vi "getIndex.vi"(11 "ModbusBuffer in":refnum<class "ModbusBuffer.lvclass">) -> (2 "Index":i32, 3 "ModbusBuffer out":refnum<class "ModbusBuffer.lvclass">)   [LabVIEW 2016, in "RTModbus.lvlib" / "ModbusBuffer.lvclass"]
uses:
  ModbusBuffer.lvclass
  ModbusBuffer.lvclass/ModbusBuffer.ctl
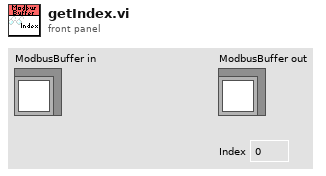
[diagram p1: front panel]
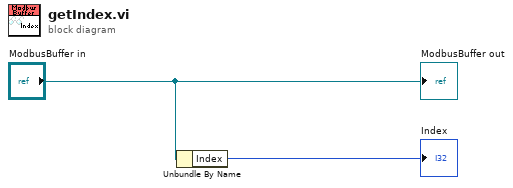
[diagram p0: block diagram]
diagram:
  n1 = Unbundle By Name("ModbusBuffer in") -> ("Index"=→"Index":i32)
  "ModbusBuffer out" <- "ModbusBuffer in"
